vi "Word_Page_Setup.vi"(0 "Word._Document":refnum<k7>, 7 "margins (1.00)":T1 {"bottom" format="%.2f"; "right" format="%.2f"; "left" format="%.2f"; "top" format="%.2f"}, 9 "measurement system (Default)":u16, 11 "error in":errorcluster) -> (8 "page width":sgl format="%.2f", 15 "error out":errorcluster)   [LabVIEW 2017, in "NI_ReportGenerationToolkit.lvlib"]
uses:
  <vilib>/addons/_office/NI_ReportGenerationToolkit.lvlib
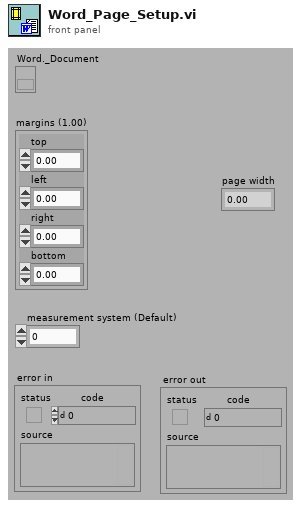
[diagram p1: front panel]
types:
  T1 = cluster{"top":dbl, "left":dbl, "right":dbl, "bottom":dbl}
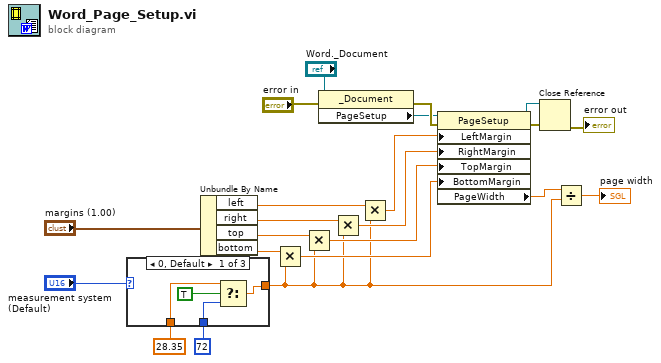
[diagram p0: block diagram]
diagram:
  n1 = case shown="0, Default" "measurement system (Default)" {
    tunnel: [w26 w27 w28] -> w1
    tunnel: 72 -> [w24 w27 _]
    tunnel: 28.35 -> [w25 _ w28]
    frame 0, Default {
      n2 = Select(t=w25, s=TRUE, f=w24) -> (s? t:f=w26:dbl)
    }
    frame 1 {
    }
    frame 2 {
    }
  }
  n3 = Unbundle By Name("margins (1.00)") -> ("left"=w21:dbl, "right"=w20:dbl, "top"=w19:dbl, "bottom"=w18:dbl)
  n4 = Multiply(x=w18, y=w1) -> (x*y=w12:dbl)
  n5 = Multiply(x=w19, y=w1) -> (x*y=w11:dbl)
  n6 = property class="_Document"(reference="Word._Document", error in="error in") -> (error out=w7:errorcluster, "PageSetup"=w4:refnum<k7>)  [unwired: 1 out]
  n7 = Multiply(x=w20, y=w1) -> (x*y=w10:dbl)
  n8 = Multiply(x=w21, y=w1) -> (x*y=w9:dbl)
  n9 = property class="PageSetup"(reference=w4, error in=w7, "LeftMargin"=w9, "RightMargin"=w10, "TopMargin"=w11, "BottomMargin"=w12) -> (reference out=w5:refnum<k7>, error out=w6:errorcluster, "PageWidth"=w2:sgl)
  n10 = Close Reference(reference=w5, error in (no error)=w6) -> (error out=→"error out":errorcluster)
  n11 = Divide(x=w2, y=w1) -> (x/y=→"page width":dbl)
